vi "PWM Loop.vi"(9 "generate pulse (T)":bool=TRUE, 10 "PWM":T1={"period (uSec)"=20000, "pulse width (uSec)"=1500}, 11 "FPGA I/O":refnum<k21>="Port1/DIO0") -> ()   [LabVIEW 2017, in "NI_Robotics_Starter Kit FPGA.lvlib"]
uses:
  <vilib>/robotics/Starter Kit/FPGA Source/NI_Robotics_Starter Kit FPGA.lvlib
  <vilib>/robotics/Utilities/FPGA Utilities/NI_Robotics_FPGA Utilities.lvlib
  <vilib>/robotics/Utilities/FPGA Utilities/Generate Digital Pulse (uSec).vi
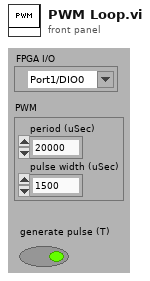
[diagram p1: front panel]
types:
  T1 = cluster{"period (uSec)":u32, "pulse width (uSec)":u32}
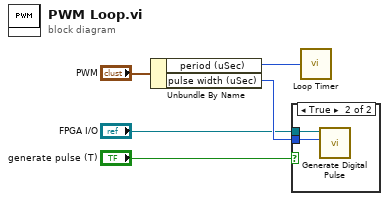
[diagram p0: block diagram]
diagram:
  n1 = Unbundle By Name("PWM") -> ("period (uSec)"=w4:u32, "pulse width (uSec)"=w3:u32)
  n2 = case shown="True" "generate pulse (T)" {
    tunnel: w3 -> [_ w7]
    tunnel: "FPGA I/O" -> [_ w6]
    frame False {
    }
    frame True {
      n3 = call-poly <vilib>:"Generate Digital Pulse.vi"("pulse width (uSec)"=w7, "FPGA digital output"=w6) -> ()  [unwired: 10 in]
    }
  }
  n4 = call "Loop Timer"("Count(uSec)"=w4) -> ()  [unwired: 1 out]
